vi "CRYOpen VI Window.vi"(10 "options":i32, 11 "WindowType":string="DockState") -> (3 "VI Ref Out":refnum<vi>)   [LabVIEW 2013]
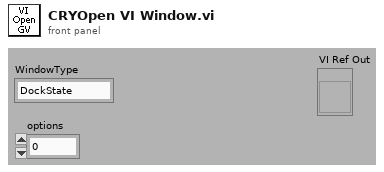
[diagram p1: front panel]
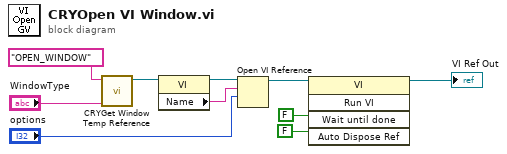
[diagram p0: block diagram]
diagram:
  n1 = call "CRYGet Window Temp Reference.vi"("sWindowName"="WindowType", "sAction"="OPEN_WINDOW") -> ("pVIRef_Out"=w6:refnum<vi>)  [unwired: 2 in, 7 out]
  n2 = property class="VI"(reference=w6) -> (reference out=w8:refnum<vi>, "Name"=w7:string)  [unwired: 1 in, 1 out]
  n3 = Open VI Reference(type specifier VI Refnum (for type only)=w8, vi path=w7, options="options") -> (vi reference=w10:refnum<vi>)  [unwired: 1 in, 3 out]
  n4 = invoke class="VI" method="Run VI"(reference=w10, "Wait until done"=FALSE ("Wait Until Done"), "Auto Dispose Ref"=FALSE ("Auto Dispose Reference")) -> (reference out=→"VI Ref Out":refnum<vi>)  [unwired: 2 in, 4 out]
